vi "声强衰减系数m计算.vi"(11 "输入频率":dbl[](array[numeric])) -> (2 "声强衰减系数m2":dbl[](array[numeric]), 3 "声强衰减系数m1":dbl[](array[numeric]))   [LabVIEW 2020]
uses:
  setup/support/rev_setup.lvlib
panel:
  out "水蒸气克分子浓度h 2":dbl
  out "氧驰豫频率frO 2":dbl
  out "氮驰豫频率frN 2":dbl
  out "大气吸收衰减系数 a2":dbl[](array[numeric])
  out "大气吸收衰减系数a":dbl[](array[numeric])
  out "氮驰豫频率frN":dbl
  out "氧驰豫频率frO":dbl
  out "水蒸气克分子浓度h":dbl
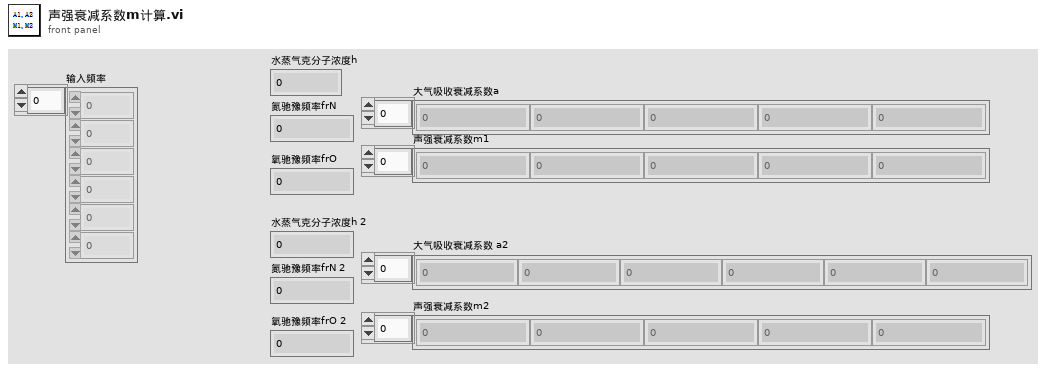
[diagram p1: front panel]
types:
  T1 = typedef "rev_setup.lvlib/EMdata.ctl" = cluster{"大气压力(kPa)":dbl, "大气压力(kPa) 2":dbl, "相对湿度(%)":dbl, "相对湿度(%)2":dbl, "大气温度(℃)":dbl, "大气温度(℃)2":dbl, "声速(m/s)":dbl, "声速(kPa)2":dbl, "混响室容积(立方米) ":dbl, "试件面积(平方米)，S":dbl, "分立吸声体个数，n":dbl}
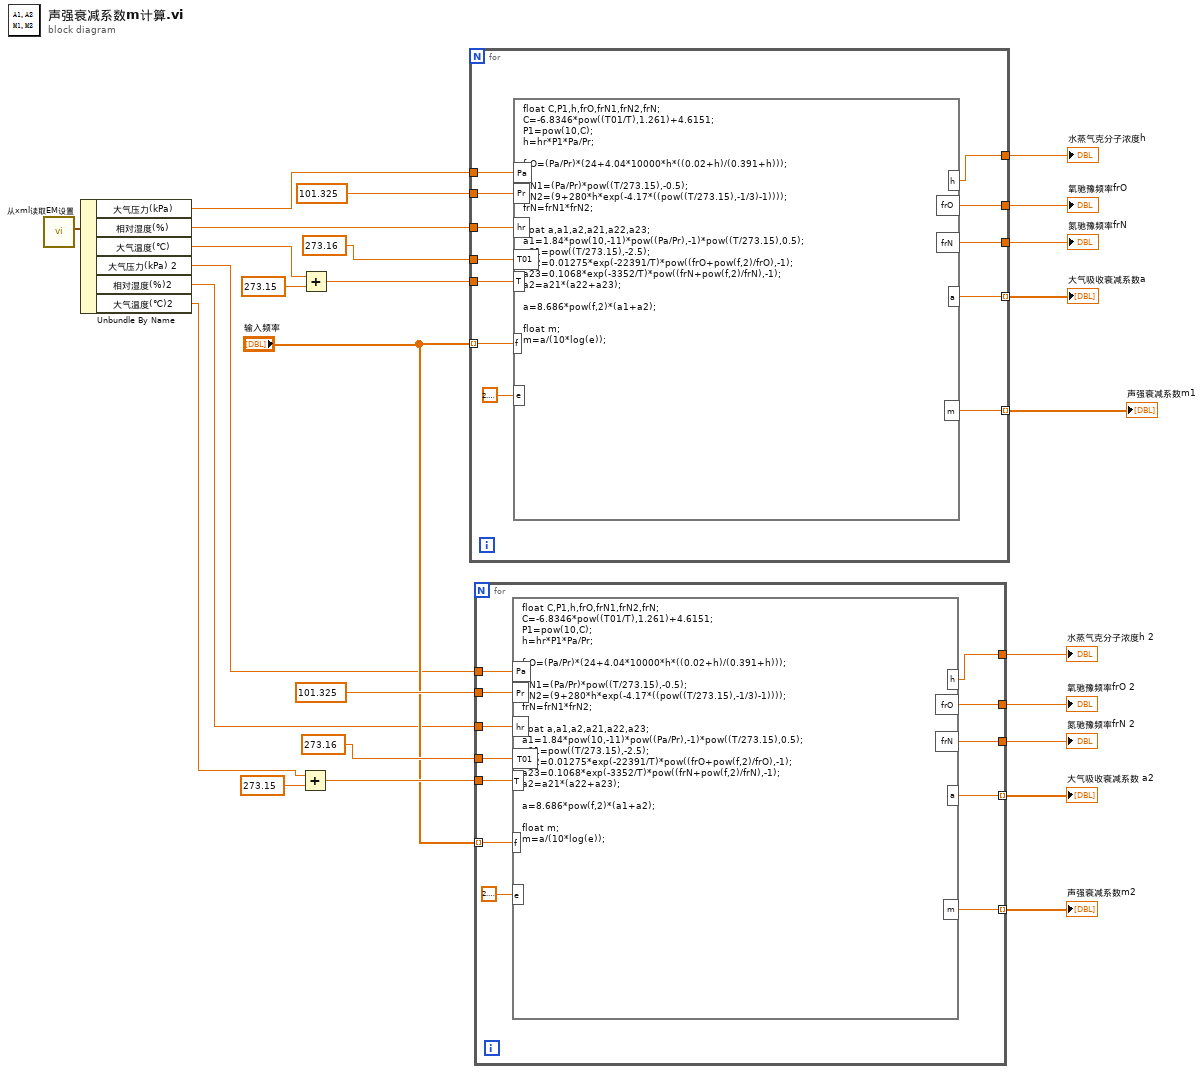
[diagram p0: block diagram]
diagram:
  n1 = call "从xml读取EM设置.vi"() -> ("EM data"=w26:T1)  [unwired: 11 in]
  n2 = Unbundle By Name(w26) -> ("大气压力(kPa)"=w20:dbl, "相对湿度(%)"=w21:dbl, "大气温度(℃)"=w24:dbl, "大气压力(kPa) 2"=w3:dbl, "相对湿度(%)2"=w2:dbl, "大气温度(℃)2"=w1:dbl)
  n3 = Add(x=w1, y=273.15) -> (x+y=w7:dbl)
  n4 = Add(x=w24, y=273.15) -> (x+y=w22:dbl)
  n5 = for {
    tunnel: 273.16 ("输入变量") -> [w38]
    tunnel: w22 -> [w37]
    tunnel: w21 -> [w36]
    tunnel: w20 -> [w35]
    tunnel: 101.325 ("输入变量") -> [w34]
    tunnel: [w33] -> w18
    tunnel: [w32] -> w17
    tunnel: [w31] -> w16
    tunnel: [w29] -> w15 mode=indexing
    tunnel: [w28] -> w14 mode=indexing
    tunnel: "输入频率" -> [w27] mode=indexing
    n6 = formula code="float C,P1,h,frO,frN1,frN2,frN;\nC=-6.8346*pow((T01/T),1.261)+4.6151;\nP1=pow(10,C);\nh=hr*P1*Pa/Pr;\n\nfrO=(Pa/Pr)*(24+4.04*10000*h*((0.02+h)/(0.391+h)));\n\nfrN1=(Pa/Pr)*pow((T/273.15),-0.5);\nfrN2=(9+280*h*exp(-4.17*((pow((T/273.15),-1/3)-1))));\nfrN=frN1*frN2;\n\nfloat a,a1,a2,a21,a22,a23;\na1=1.84*pow(10,-11)*pow((Pa/Pr),-1)*pow((T/273.15),0.5);\na21=pow((T/273.15),-2.5);\na22=0.01275*exp(-22391/T)*pow((frO+pow(f,2)/frO),-1);\na23=0.1068*exp(-3352/T)*pow((frN+pow(f,2)/frN),-1);\na2=a21*(a22+a23);\n\na=8.686*pow(f,2)*(a1+a2);\n\nfloat m;\nm=a/(10*log(e));"("T01"=w38, "T"=w37, "hr"=w36, "Pa"=w35, "Pr"=w34, "f"=w27, "e"=2.718281828459045) -> ("h"=w33:dbl, "frO"=w32:dbl, "frN"=w31:dbl, "m"=w28:dbl, "a"=w29:dbl)
  }
  "水蒸气克分子浓度h" <- w18
  "氧驰豫频率frO" <- w17
  "氮驰豫频率frN" <- w16
  "大气吸收衰减系数a" <- w15
  "声强衰减系数m1" <- w14
  n7 = for {
    tunnel: [w50] -> w13 mode=indexing
    tunnel: [w49] -> w12 mode=indexing
    tunnel: [w47] -> w11
    tunnel: [w46] -> w10
    tunnel: [w45] -> w9
    tunnel: 101.325 ("输入变量") -> [w44]
    tunnel: w7 -> [w43]
    tunnel: 273.16 ("输入变量") -> [w42]
    tunnel: "输入频率" -> [w41] mode=indexing
    tunnel: w3 -> [w40]
    tunnel: w2 -> [w39]
    n8 = formula code="float C,P1,h,frO,frN1,frN2,frN;\nC=-6.8346*pow((T01/T),1.261)+4.6151;\nP1=pow(10,C);\nh=hr*P1*Pa/Pr;\n\nfrO=(Pa/Pr)*(24+4.04*10000*h*((0.02+h)/(0.391+h)));\n\nfrN1=(Pa/Pr)*pow((T/273.15),-0.5);\nfrN2=(9+280*h*exp(-4.17*((pow((T/273.15),-1/3)-1))));\nfrN=frN1*frN2;\n\nfloat a,a1,a2,a21,a22,a23;\na1=1.84*pow(10,-11)*pow((Pa/Pr),-1)*pow((T/273.15),0.5);\na21=pow((T/273.15),-2.5);\na22=0.01275*exp(-22391/T)*pow((frO+pow(f,2)/frO),-1);\na23=0.1068*exp(-3352/T)*pow((frN+pow(f,2)/frN),-1);\na2=a21*(a22+a23);\n\na=8.686*pow(f,2)*(a1+a2);\n\nfloat m;\nm=a/(10*log(e));"("T01"=w42, "T"=w43, "hr"=w39, "Pa"=w40, "Pr"=w44, "f"=w41, "e"=2.718281828459045) -> ("h"=w45:dbl, "frO"=w46:dbl, "frN"=w47:dbl, "m"=w50:dbl, "a"=w49:dbl)
  }
  "水蒸气克分子浓度h 2" <- w9
  "氧驰豫频率frO 2" <- w10
  "氮驰豫频率frN 2" <- w11
  "大气吸收衰减系数 a2" <- w12
  "声强衰减系数m2" <- w13
